vi "GetImageMaxMinMedian.vi"(11 "Image":u16[][](array[numeric])) -> (1 "Max":u16, 2 "Median":u16, 3 "Min":u16)   [LabVIEW 2017]
uses:
  <userlib>/_OpenG.lib/array/array.llb/Sort 1D Array (U16)__ogtk.vi
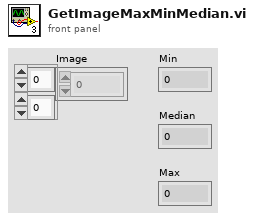
[diagram p1: front panel]
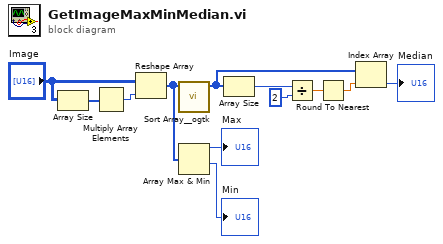
[diagram p0: block diagram]
diagram:
  n1 = Array Size(array="Image") -> (size(s)=w2:i32[])
  n2 = Multiply Array Elements(1:w2) -> (0:w1:i32)
  n3 = Reshape Array("Image", w1) -> (w6:u16[])
  n4 = call-poly <userlib>:"Sort Array__ogtk.vi"("Array in"=w6) -> ("Sorted Array out"=w7:u16[])  [unwired: 9 in, 1 out]
  n5 = Array Max & Min(array=w6) -> (max value=→"Max":u16, min value=→"Min":u16)  [unwired: 2 out]
  n6 = Array Size(array=w7) -> (size(s)=w8:i32)
  n7 = Divide(x=w8, y=2) -> (x/y=w11:dbl)
  n8 = Round To Nearest(number=w11) -> (nearest integer value=w12:dbl)
  n9 = Index Array(array=w7, index=w12) -> (element=→"Median":u16)
